vi "InventoryManager_ManualUpdate--UI.vi"(8 "error In":errorcluster) -> (0 "error Out":errorcluster)   [LabVIEW 2020]
uses:
  BRS_Dev/Source Code/Inventory Manager/Controls/IM_Cluster.ctl
  BRS_Dev/Source Code/Inventory Manager/Controls/IM_Options.ctl
  BRS_Dev/Source Code/Inventory Manager/Controls/IM_Result.ctl
  BRS_Dev/Source Code/Database/DB Driver/BRS_DB Driver Main Options.ctl
  BRS_Dev/Source Code/Database/DB Driver/DB functions in.ctl
  <vilib>/Utility/NIReport.llb/NI_report.lvclass
  BRS_Dev/Source Code/Utility/Global.vi
  BRS_Dev/Source Code/Global/Global 1.vi
panel:
  in  "Search Option":T1 {"Module" max=114; "Column" max=12; "Row" max=114; "Stocker" items=["Stocker Left", "Stocker Center", "Stocker Right"]}
  in  "Reticle ID":string
  in  "Import Inven_XL":bool
  out "Reset":T2 {"Location status" items=["Disabled/Unusable  ", "Empty ", "Full  "]}
  in  "Exit":bool
  in  "Result":T2 {"Location status" items=["Disabled/Unusable  ", "Empty ", "Full  "]}
  in  "Search":bool
  out "Status":string
  in  "Reset":bool
  out "Date and Time :":string
  in  "Update":bool
  # "Inventory Manager"
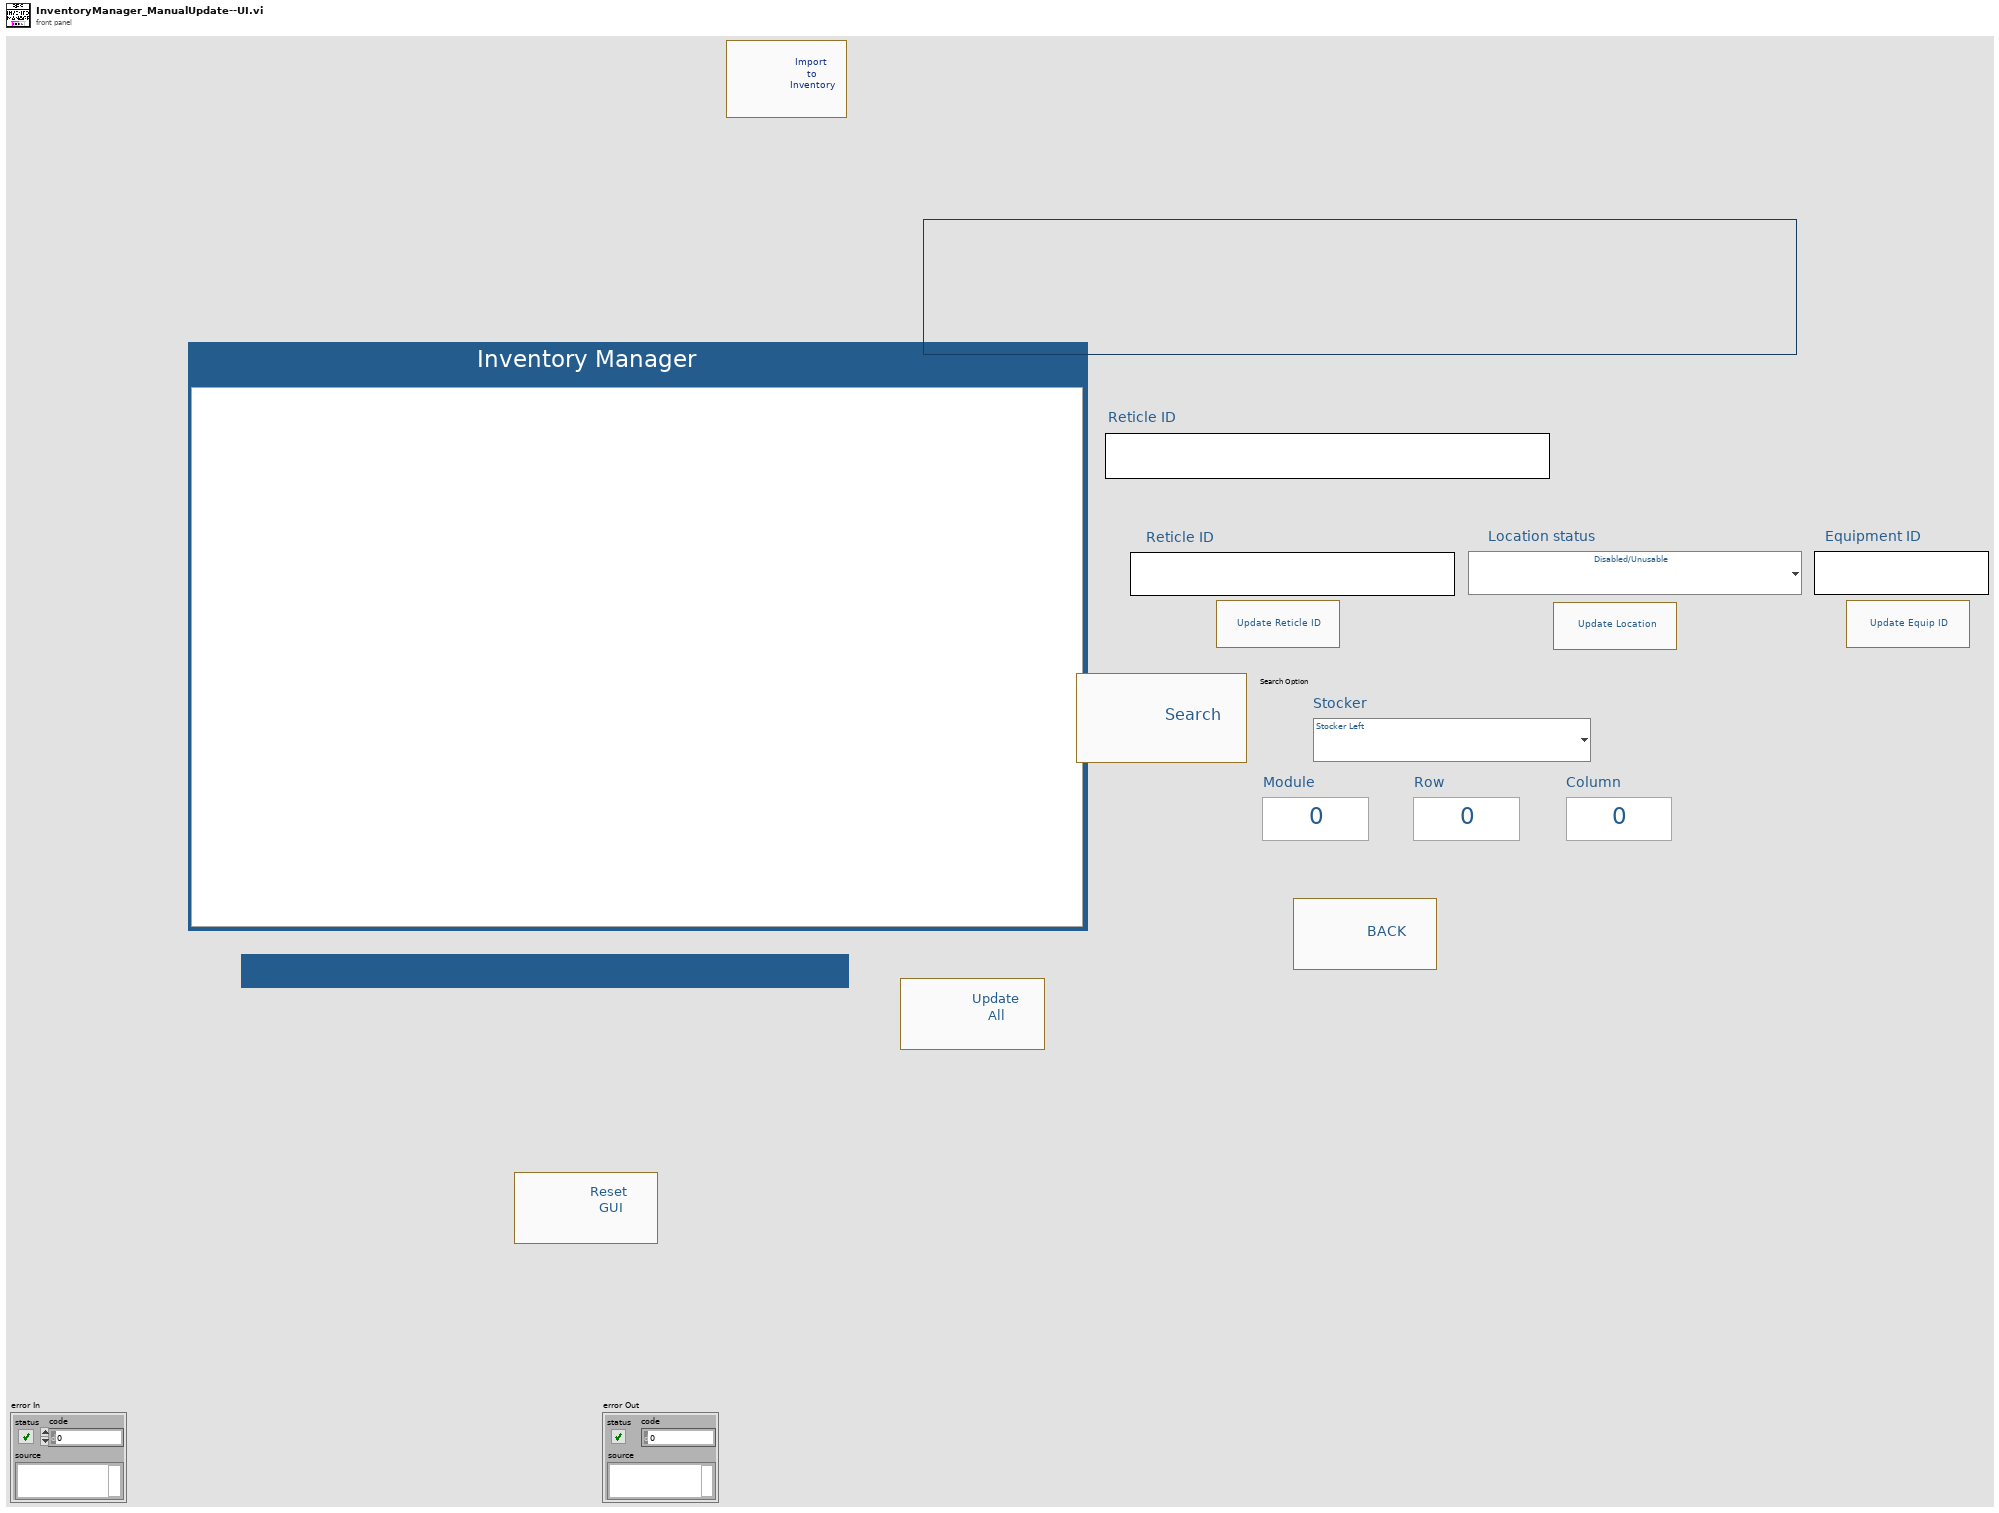
[diagram p1: front panel]
types:
  T1 = typedef "IM_Cluster.ctl" = cluster{"Stocker":u16, "Row":u16, "Column":u16, "Module":u16}
  T2 = typedef "IM_Result.ctl" = cluster{"Location status":u16, "Reticle ID":string, "Equipment ID":string, "Ret_Update":bool, "Loc_Update":bool, "Eqp_Update":bool}
  T3 = typedef "IM_Options.ctl" = enum16{"Poll", "Init", "Update DB", "Reset", "Search", "Error", "Exit"}
  T4 = typedef "LVRectTypeDef.ctl" = cluster{"Left":i16, "Top":i16, "Right":i16, "Bottom":i16}
  T5 = typedef "Basic FP Settings--cluster.ctl" = cluster{"Front Panel.Closeable":bool, "Front Panel.Minimizeable":bool, "Front Panel.Resizeable":bool, "Front Panel.ShowMenuBar":bool, "Front Panel.TitleBarVis":bool, "TB.Visible":bool, "Horizontal Scrollbar Visibility":enum16{"Always On", "Always Off", "Off While Running"}, "Vertical Scrollbar Visibility":enum16{"Always On", "Always Off", "Off While Running"}}
  T6 = enum16{"maximized", "minimized", "normal", "no change"}
  T7 = enum16{"Standard Report", "HTML", "Word", "Excel"}
  T8 = enum32{"Stocker", "Reticle ID", "Multiple Inventory Update"}
  T9 = typedef "DB functions in.ctl" = cluster{"Order By":string, "Where":string, "Table /DBName/Query":string, "Values":string[], "Column Names":string[], "Where_Multi Colum":string[], "Where_Multi Value":string[]}
  T10 = typedef "BRS_DB Driver Main Options.ctl" = enum16{"Open", "RefOut", "Select", "Execute", "Update Multi", "Update Single", "Update Multi Column", "Insert", "Insert OrUpdate", "Delete", "Close"}
  T11 = typedef "DB functions outs.ctl" = cluster{"Selected Data":string[][], "Element":string, "First Slot":string[], "Response":T12}
  T12 = typedef "Q Msgs.ctl" = enum16{"FINISHED", "ABORT", "READY", "COMMUNICATION ERROR", "SCAN PROGRESS", "CHANGE LOCATION", "POS REACHED", "HOME REACHED", "ERROR", "PDS HOME", "PDS ERROR", "PDS STATUS", "PDS START", "PDS ABORT", "PDS PASS", "PDS FAIL", "PDS Recipe", "NONE", "RC START", "RC REACHED", "RC COMPLETED", "START SCAN", "VACC_ERROR", "MLP RET PRES ERROR", "MLP DOOR ERROR", "MLP OK", "MLP FINISHED", "MLP POD CAPT ERROR", "MLP LID CAPT ERROR", "MLP OPEN CYL  ERROR", "MLP CLOSE CYL ERROR", "MLP POD PRE ERROR", "MLP POD UNLATCHED", "RC TOP", "RC BOTTOM", "EXIT"}
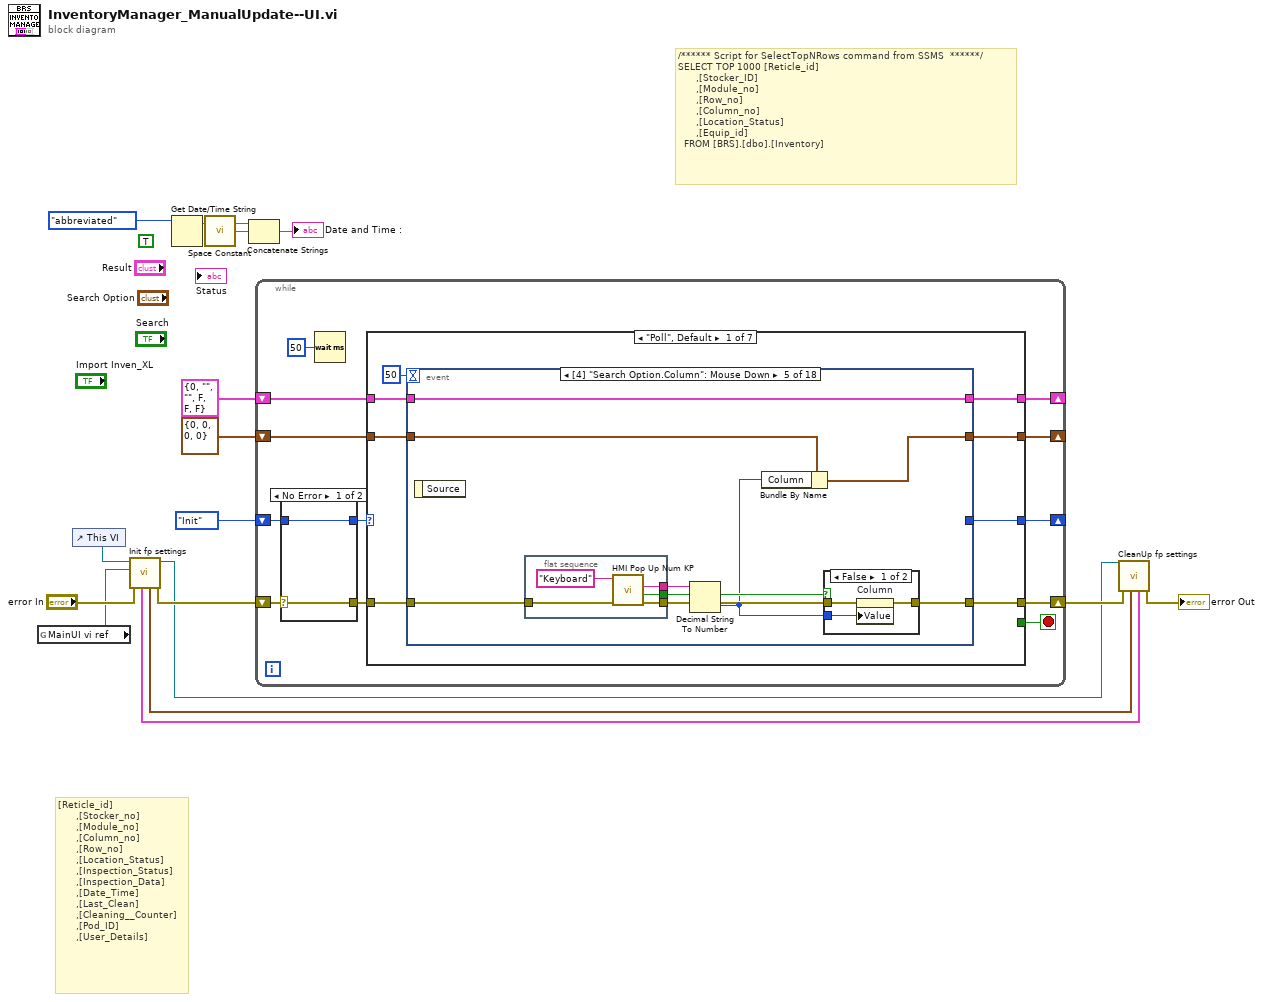
[diagram p0: block diagram]
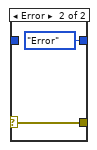
[diagram p2: hidden frame]
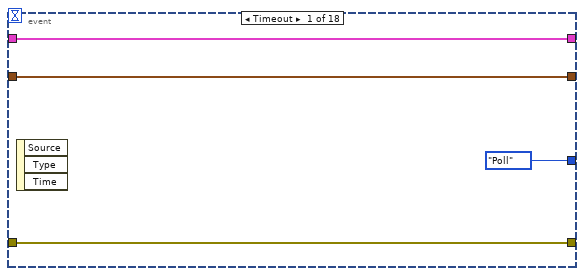
[diagram p3: hidden frame]
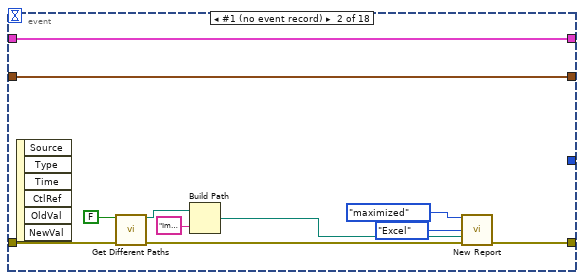
[diagram p4: hidden frame]
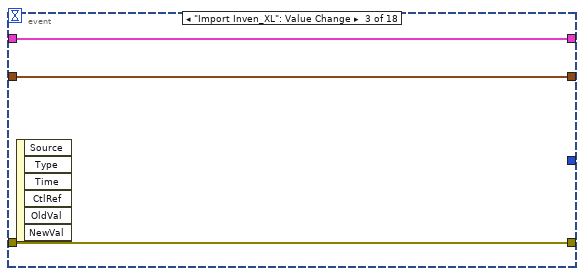
[diagram p5: hidden frame]
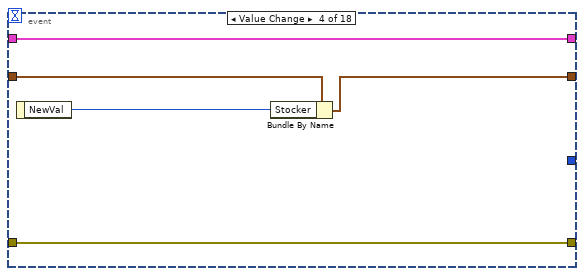
[diagram p6: hidden frame]
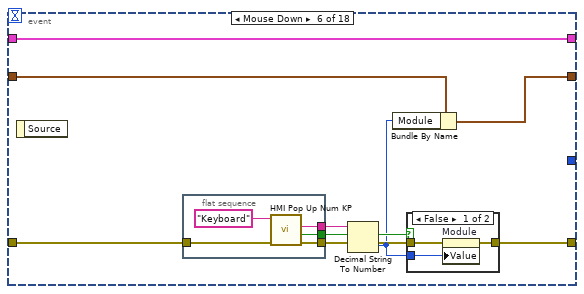
[diagram p8: hidden frame]
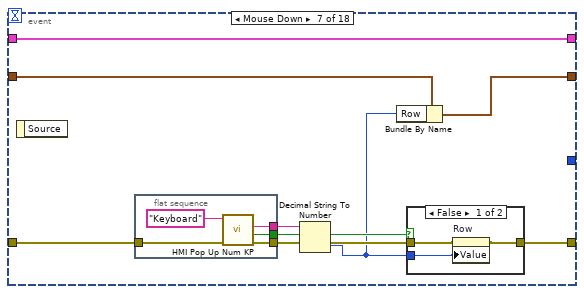
[diagram p10: hidden frame]
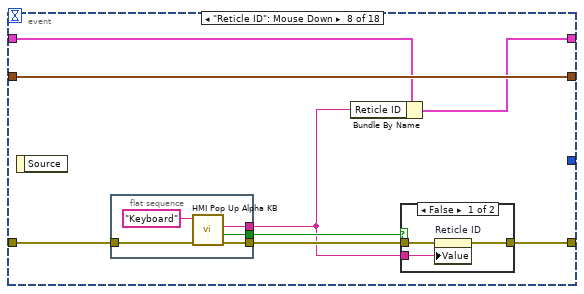
[diagram p12: hidden frame]
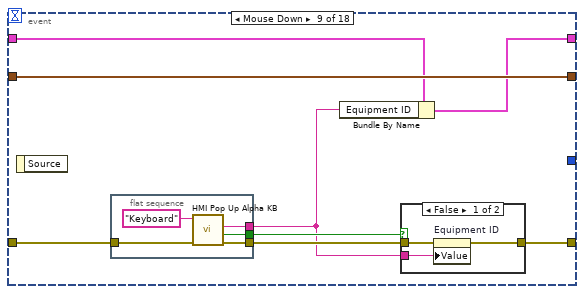
[diagram p14: hidden frame]
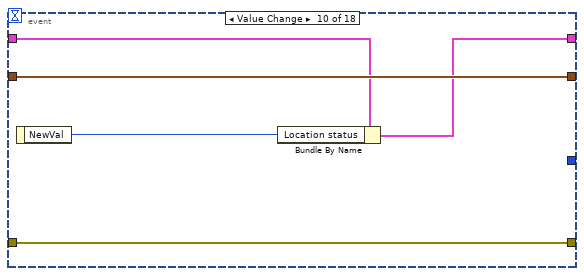
[diagram p16: hidden frame]
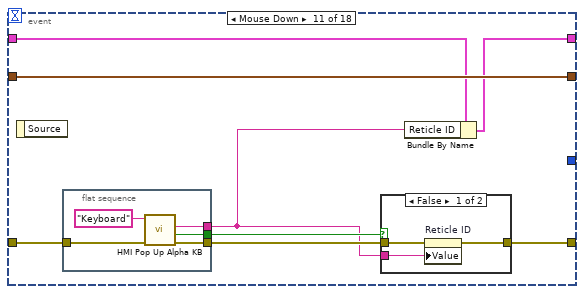
[diagram p17: hidden frame]
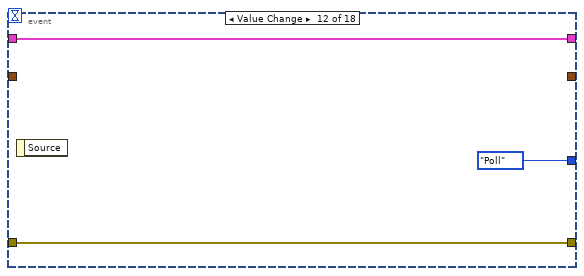
[diagram p19: hidden frame]
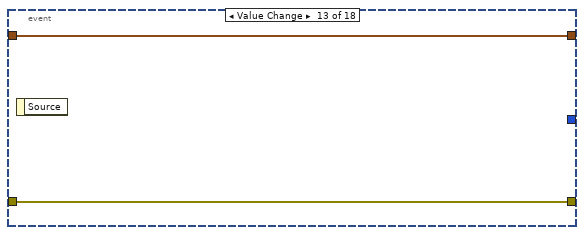
[diagram p20: hidden frame]
diagram:
  (unwired) TRUE ("want seconds? (F)")
  # "/****** Script for SelectTopNRows command from SSMS  ******/\nSELECT TOP 1000 [Reticle_id]\n      ,[Stocker_ID]\n      ,[Module_no]\n      ,[Row_no]\n      ,[Column_no]\n      ,[Location_Status]\n      ,[Equip_id]\n  FROM [BRS].[dbo].[Inventory]"
  # "[Reticle_id]\n      ,[Stocker_no]\n      ,[Module_no]\n      ,[Column_no]\n      ,[Row_no]\n      ,[Location_Status]\n      ,[Inspection_Status]\n      ,[Inspection_Data]\n      ,[Date_Time]\n      ,[Last_Clean]\n      ,[Cleaning__Counter]\n      ,[Pod_ID]\n      ,[User_Details]"
  n1 = global read "Global 1.vi" "MainUI vi ref"() -> (w5:refnum<vi>)
  n2 = control-ref of="This VI"() -> (w13:refnum<vi>)
  n3 = call "Init fp settings.vi"("error in (no error)"="error In", "Caller VI Refnum (Callee's Caller)"=w5, "vi reference"=w13) -> ("error out"=w9:errorcluster, "vi reference out"=w6:refnum<vi>, "Front Panel Window:Panel Bounds"=w8:T4, "Original basic fp settings"=w7:T5)  [unwired: 3 in]
  n4 = Get Date/Time String(date format (0)=enum16{"short", "long", "abbreviated"}."abbreviated") -> (date string=w2:string)  [unwired: 2 in, 1 out]
  n5 = call <vilib>:"Space Constant.vi"() -> ("String"=w3:string)
  n6 = Concatenate Strings(w2, w3) -> (→"Date and Time :":string)  [unwired: 1 in]
  n7 = while {
    shift-right: [w28] -> _
    shift-left: IM_Options."Init" -> [w22]
    shift-right: [w26] -> w12
    shift-left: w9 -> [w25]
    shift-right: [w21] -> _
    shift-left: T1 {"Stocker"=0, "Row"=0, "Column"=0, "Module"=0} ("Clean Loc") -> [w20]
    shift-right: [w19] -> _
    shift-left: T2 {"Location status"=0, "Reticle ID"="", "Equipment ID"="", "Ret_Update"=FALSE, "Loc_Update"=FALSE, "Eqp_Update"=FALSE} ("Result") -> [w18]
    stop <- w27 stop-if-true
    n8 = case shown="No Error" w25 {
      selector: w25 -> [w30 w31]
      tunnel: [w30 w31] -> w24
      tunnel: [w29 IM_Options."Error"] -> w23
      tunnel: w22 -> [w29 _]
      frame No Error {
      }
      frame Error {
      }
    }
    n9 = Wait (ms)(milliseconds to wait=u32 50) -> ()  [unwired: 1 out]
    n10 = case shown="\"Poll\", Default" w23 {
      tunnel: [w39 IM_Options."Poll" IM_Options."Poll" IM_Options."Poll" IM_Options."Poll" IM_Options."Poll" IM_Options."Poll"] -> w28
      tunnel: [_ _ _ _ _ _ TRUE] -> w27
      tunnel: [w38 w225 w230 w235 w244 w270 w280] -> w26
      tunnel: w24 -> [w37 w223 _ w235 w247 w272 w280]
      tunnel: [w36 w226 w232 w236 w242 w274 w278] -> w21
      tunnel: w20 -> [w35 w226 w232 w236 w242 w274 w278]
      tunnel: [w33 _ w229 w234 w238 w273 w277] -> w19
      tunnel: w18 -> [w34 _ w231 _ _ w273 w277]
      frame "Poll", Default {
        n11 = event shown="[4] \"Search Option.Column\": Mouse Down" {
          selector: _ -> [_ _ _ _ _ _ _ _ _ _ _ _ _ _ _ _ _ _]
          dyn-events: _ -> [_ _ _ _ _ _ _ _ _ _ _ _ _ _ _ _ _ _]
          timeout: 50 -> [_ _ _ _ _ _ _ _ _ _ _ _ _ _ _ _ _ _]
          tunnel: [IM_Options."Poll" _ _ _ _ _ _ _ _ _ _ IM_Options."Poll" _ IM_Options."Search" w190 _ IM_Options."Reset" IM_Options."Exit"] -> w39
          tunnel: [w43 w45 w56 w63 w67 w85 w103 w121 w138 w156 w160 w176 w178 w182 w192 w195 w216 w220] -> w38
          tunnel: w37 -> [w43 w46 w56 w63 w71 w89 w107 w124 w141 w156 w163 w176 w178 w182 w192 w194 w216 w220]
          tunnel: [w42 w55 w58 w60 w65 w83 w101 w125 w142 w155 w164 _ w177 w181 w191 w197 w215 w219] -> w36
          tunnel: w35 -> [w42 w55 w58 w61 w66 w84 w102 w125 w142 w155 w164 _ w177 w181 w191 _ w215 w219]
          tunnel: w34 -> [w41 w54 w57 w62 w72 w90 w108 w120 w137 w154 w159 w174 _ w179 _ _ w214 w218]
          tunnel: [w41 w54 w57 w62 w72 w90 w108 w119 w136 w153 w158 w174 _ w179 w183 w198 w214 w218] -> w33
          event Timeout {
            n12 = event-data() -> ()  [unwired: 1 in, 3 out]
          }
          event #1 (no event record) {
            n13 = event-data() -> ()  [unwired: 1 in, 6 out]
            n14 = call "Get Different Paths.vi"("Initialize(Default: Off)"=FALSE, "error in"=w46) -> ("Info File Path"=w48:path, "error out"=w53:errorcluster)  [unwired: 7 in, 5 out]
            n15 = Build Path(base path=w48, name or relative path="Import Inventory Templete.xlt") -> (appended path=w52:path)
            n16 = call <vilib>:"New Report.vi"("window state (normal)"=T6."maximized", "report type"=T7."Excel", "template (empty)"=w52, "error in (no error)"=w53) -> ("error out"=w45:errorcluster)  [unwired: 10 in, 1 out]
          }
          event "Import Inven_XL": Value Change {
            n17 = event-data() -> ()  [unwired: 1 in, 6 out]
          }
          event Value Change {
            n18 = event-data() -> ("NewVal"=w59:u16)  [unwired: 1 in]
            n19 = Bundle By Name(cluster=w61, "Stocker"=w59) -> (w60:T1)
          }
          event Mouse Down {
            n20 = event-data() -> ()  [unwired: 1 in, 1 out]
            n21 = flat-sequence {
              tunnel: [w77] -> w68
              tunnel: w71 -> [w78]
              tunnel: [w80] -> w70
              tunnel: [w79] -> w69
              frame #0 {
                n22 = call "HMI Pop Up Num KP.vi"("error in"=w78, "Message In"="Keyboard") -> ("error out"=w77:errorcluster, "Canceled"=w79:bool, "String Out"=w80:string)  [unwired: 7 in]
              }
            }
            n23 = Decimal String To Number(string=w70) -> (number=w64:i32)  [unwired: 2 in, 1 out]
            n24 = Bundle By Name(cluster=w66, "Column"=w64) -> (w65:T1)
            n25 = case shown="False" w69 {
              tunnel: w64 -> [w75 _]
              tunnel: w68 -> [w74 w76]
              tunnel: [w73 w76] -> w67
              frame False {
                n26 = property on="Column" class="DigNum (strict)"(error in=w74, "Value"=w75) -> (error out=w73:errorcluster)  [unwired: 1 in, 1 out]
              }
              frame True {
              }
            }
          }
          event Mouse Down {
            n27 = event-data() -> ()  [unwired: 1 in, 1 out]
            n28 = flat-sequence {
              tunnel: [w95] -> w86
              tunnel: w89 -> [w96]
              tunnel: [w98] -> w88
              tunnel: [w97] -> w87
              frame #0 {
                n29 = call "HMI Pop Up Num KP.vi"("error in"=w96, "Message In"="Keyboard") -> ("error out"=w95:errorcluster, "Canceled"=w97:bool, "String Out"=w98:string)  [unwired: 7 in]
              }
            }
            n30 = Decimal String To Number(string=w88) -> (number=w82:i32)  [unwired: 2 in, 1 out]
            n31 = Bundle By Name(cluster=w84, "Module"=w82) -> (w83:T1)
            n32 = case shown="False" w87 {
              tunnel: w82 -> [w93 _]
              tunnel: w86 -> [w92 w94]
              tunnel: [w91 w94] -> w85
              frame False {
                n33 = property on="Module" class="DigNum (strict)"(error in=w92, "Value"=w93) -> (error out=w91:errorcluster)  [unwired: 1 in, 1 out]
              }
              frame True {
              }
            }
          }
          event Mouse Down {
            n34 = event-data() -> ()  [unwired: 1 in, 1 out]
            n35 = flat-sequence {
              tunnel: [w113] -> w104
              tunnel: w107 -> [w114]
              tunnel: [w116] -> w106
              tunnel: [w115] -> w105
              frame #0 {
                n36 = call "HMI Pop Up Num KP.vi"("error in"=w114, "Message In"="Keyboard") -> ("error out"=w113:errorcluster, "Canceled"=w115:bool, "String Out"=w116:string)  [unwired: 7 in]
              }
            }
            n37 = Decimal String To Number(string=w106) -> (number=w100:i32)  [unwired: 2 in, 1 out]
            n38 = Bundle By Name(cluster=w102, "Row"=w100) -> (w101:T1)
            n39 = case shown="False" w105 {
              tunnel: w100 -> [w109 _]
              tunnel: w104 -> [w111 w112]
              tunnel: [w110 w112] -> w103
              frame False {
                n40 = property on="Row" class="DigNum (strict)"(error in=w111, "Value"=w109) -> (error out=w110:errorcluster)  [unwired: 1 in, 1 out]
              }
              frame True {
              }
            }
          }
          event "Reticle ID": Mouse Down {
            n41 = event-data() -> ()  [unwired: 1 in, 1 out]
            n42 = flat-sequence {
              tunnel: [w130] -> w122
              tunnel: w124 -> [w131]
              tunnel: [w133] -> w118
              tunnel: [w132] -> w123
              frame #0 {
                n43 = call "HMI Pop Up Alpha KB.vi"("error in"=w131, "Message In"="Keyboard") -> ("error out"=w130:errorcluster, "Canceled"=w132:bool, "String Out"=w133:string)  [unwired: 7 in]
              }
            }
            n44 = Bundle By Name(cluster=w120, "Reticle ID"=w118) -> (w119:T2)
            n45 = case shown="False" w123 {
              tunnel: w118 -> [w128 _]
              tunnel: w122 -> [w127 w129]
              tunnel: [w126 w129] -> w121
              frame False {
                n46 = property on="Reticle ID" class="Str"(error in=w127, "Value"=w128) -> (error out=w126:errorcluster)  [unwired: 1 in, 1 out]
              }
              frame True {
              }
            }
          }
          event Mouse Down {
            n47 = event-data() -> ()  [unwired: 1 in, 1 out]
            n48 = flat-sequence {
              tunnel: [w147] -> w139
              tunnel: w141 -> [w148]
              tunnel: [w150] -> w135
              tunnel: [w149] -> w140
              frame #0 {
                n49 = call "HMI Pop Up Alpha KB.vi"("error in"=w148, "Message In"="Keyboard") -> ("error out"=w147:errorcluster, "Canceled"=w149:bool, "String Out"=w150:string)  [unwired: 7 in]
              }
            }
            n50 = Bundle By Name(cluster=w137, "Equipment ID"=w135) -> (w136:T2)
            n51 = case shown="False" w140 {
              tunnel: w135 -> [w144 _]
              tunnel: w139 -> [w145 w146]
              tunnel: [w143 w146] -> w138
              frame False {
                n52 = property on="Equipment ID" class="Str"(error in=w145, "Value"=w144) -> (error out=w143:errorcluster)  [unwired: 1 in, 1 out]
              }
              frame True {
              }
            }
          }
          event Value Change {
            n53 = event-data() -> ("NewVal"=w152:u16)  [unwired: 1 in]
            n54 = Bundle By Name(cluster=w154, "Location status"=w152) -> (w153:T2)
          }
          event Mouse Down {
            n55 = event-data() -> ()  [unwired: 1 in, 1 out]
            n56 = flat-sequence {
              tunnel: [w169] -> w161
              tunnel: w163 -> [w170]
              tunnel: [w172] -> w157
              tunnel: [w171] -> w162
              frame #0 {
                n57 = call "HMI Pop Up Alpha KB.vi"("error in"=w170, "Message In"="Keyboard") -> ("error out"=w169:errorcluster, "Canceled"=w171:bool, "String Out"=w172:string)  [unwired: 7 in]
              }
            }
            n58 = case shown="False" w162 {
              tunnel: w157 -> [w167 _]
              tunnel: w161 -> [w166 w168]
              tunnel: [w165 w168] -> w160
              frame False {
                n59 = property on="Reticle ID" class="Str"(error in=w166, "Value"=w167) -> (error out=w165:errorcluster)  [unwired: 1 in, 1 out]
              }
              frame True {
              }
            }
            n60 = Bundle By Name(cluster=w159, "Reticle ID"=w157) -> (w158:T2)
          }
          event Value Change {
            n61 = event-data() -> ()  [unwired: 1 in, 1 out]
          }
          event Value Change {
            n62 = event-data() -> ()  [unwired: 1 in, 1 out]
          }
          event "Search": Value Change {
            n63 = event-data() -> ()  [unwired: 1 in, 1 out]
          }
          event "Update": Value Change {
            n64 = event-data() -> ()  [unwired: 1 in, 1 out]
            n65 = call "Popup_Twobutton.vi"("Yes Text"="YES" ("Exit Text"), "No Text"="NO" ("Exit Text"), "Message in"="Are You Sure..\nDo you want to update Inventory??" ("message")) -> ("NoButton Pressed?"=w186:bool)  [unwired: 7 in, 1 out]
            n66 = local read "Result"() -> (w183:T2)
            n67 = Select(t=IM_Options."Poll", s=w186, f=IM_Options."Update DB") -> (s? t:f=w190:T3)
          }
          event #15 (no event record) {
            w197 = T1 {"Stocker"=0, "Row"=0, "Column"=0, "Module"=0} ("Clean Loc")
            w198 = T2 {"Location status"=0, "Reticle ID"="", "Equipment ID"="STK09601", "Ret_Update"=FALSE, "Loc_Update"=FALSE, "Eqp_Update"=FALSE} ("Result")
            n68 = event-data() -> ("NewVal"=w196)  [unwired: 1 in]
            n69 = case shown="\"Reticle ID\"" w196 {
              tunnel: w194 -> [w203 w208 w213]
              tunnel: [w201 w206 w211] -> w195
              tunnel: [w200 2 0] -> w193
              frame "Stocker", Default {
                w200 = 0
                n70 = property on="Search" class="Bool"(error in=w203, "DisabledEnum"=w200) -> (error out=w202:errorcluster)  [unwired: 1 in, 1 out]
                n71 = property on="Result" class="Clust (strict)"(error in=w202, "DisabledEnum"=w200) -> (error out=w201:errorcluster)  [unwired: 1 in, 1 out]
              }
              frame "Reticle ID" {
                w205 = 0
                n72 = property on="Search" class="Bool"(error in=w208, "DisabledEnum"=w205) -> (error out=w207:errorcluster)  [unwired: 1 in, 1 out]
                n73 = property on="Result" class="Clust (strict)"(error in=w207, "DisabledEnum"=w205) -> (error out=w206:errorcluster)  [unwired: 1 in, 1 out]
              }
              frame "Multiple Inventory Update" {
                w210 = 2
                n74 = property on="Search" class="Bool"(error in=w213, "DisabledEnum"=w210) -> (error out=w212:errorcluster)  [unwired: 1 in, 1 out]
                n75 = property on="Result" class="Clust (strict)"(error in=w212, "DisabledEnum"=w210) -> (error out=w211:errorcluster)  [unwired: 1 in, 1 out]
              }
            }
            n76 = local write "Reticle ID"("" ("Reticle ID")) -> ()
            n77 = local write "Result"(w198) -> ()
            n78 = local write "Search Option"(w197) -> ()
            n79 = property on="Eqp_Update" class="Bool (strict)"("DisabledEnum"=w193) -> ()  [unwired: 2 in, 2 out]
            n80 = property on="Ret_Update" class="Bool (strict)"("DisabledEnum"=w193) -> ()  [unwired: 2 in, 2 out]
            n81 = property on="Loc_Update" class="Bool (strict)"("DisabledEnum"=w193) -> ()  [unwired: 2 in, 2 out]
          }
          event "Reset": Value Change {
            n82 = event-data() -> ()  [unwired: 1 in, 1 out]
          }
          event "Exit": Value Change {
            n83 = event-data() -> ()  [unwired: 1 in, 6 out]
          }
        }
      }
      frame "Init" {
        n84 = global read "Global.vi" "Run?"() -> (w224:bool)
        n85 = local write item#-1(T8."Stocker" ("Inv_Manag")) -> ()
        n86 = local write "Search Option"(w226) -> ()
        n87 = local read "Status"() -> (w227:string)
      }
      frame "Update DB" {
      }
      frame "Reset" {
      }
      frame "Search" {
        n88 = case shown="\"Reticle ID\"" w246 {
          tunnel: w247 -> [w261 _]
          tunnel: [w266 _] -> w245
          tunnel: T9 {"Order By"="", "Where"="", "Table /DBName/Query"="[BRS].[dbo].[Inventory]", "Values"=[], "Column Names"=[], "Where_Multi Colum"=[], "Where_Multi Value"=[]} ("DB Fun in") -> [w264 w269]
          tunnel: [w265 _] -> w243
          tunnel: w242 -> [w262 _]
          tunnel: string[] ["Reticle_id", "Location_Status", "Equip_id"] ("Column Names") -> [w254 w268]
          tunnel: string[] ["L", "C", "R"] -> [w253 _]
          frame "Stocker", Default {
            n89 = Cluster To Array(cluster=w262) -> (array=w259:u16[])
            n90 = Index Array(array=w259) -> (element #1=w251:u16, element #2=w258:u16, element #3=w257:u16, element #4=w256:u16)  [unwired: 4 in]
            n91 = Index Array(array=w253, index=w251) -> (element=w252:string)
            n92 = Format Into String(format string="Stocker_ID='%S' and\n Row_no='%d' and Column_no='%d' and Module_no='%d' " ("string"), error in=w261, w252, w258, w257, w256) -> (resulting string=w255:string, error out=w260:errorcluster)  [unwired: 1 in]
            n93 = Bundle By Name(cluster=w264, "Column Names"=w254, "Where"=w255) -> (w263:T9)
            n94 = call "BRS_DB Driver Main.vi"("Option"=BRS_DB_Driver_Main_Options."Select", "error in (no error)"=w260, "DB Fun in"=w263) -> ("error out"=w266:errorcluster, "output cluster"=w265:T11)  [unwired: 4 in, 3 out]
          }
          frame "Reticle ID" {
          }
        }
        n95 = local write "Status"("Search Completed...." ("Status")) -> ()
        n96 = call "Selected data to cluster.vi"("error in"=w245, "output cluster in"=w243) -> ("error out"=w244:errorcluster, "output cluster out"=w238:T2)  [unwired: 8 in]
        "Reset" <- w238
        n97 = local write "Result"(w238) -> ()
      }
      frame "Error" {
        n98 = call "Error Pop.vi"("error in"=w272) -> ("error out"=w271:errorcluster)  [unwired: 10 in]
        n99 = call <vilib>:"Clear Errors.vi"("error in (no error)"=w271) -> ("error out"=w270:errorcluster)  [unwired: 5 in, 1 out]
      }
      frame "Exit" {
      }
    }
  }
  n100 = call "CleanUp fp settings.vi"("Original basic fp settings"=w7, "Front Panel Window:Panel Bounds"=w8, "error in (no error)"=w12, "vi reference"=w6) -> ("error out"=→"error Out":errorcluster)  [unwired: 4 in, 1 out]
